vi "BMU参数读取-Auto.vi"(7 "Socket":dbl, 8 "CAN端口":u16(ring), 9 "设备索引号":u16(ring), 10 "CAN卡类型":u32(ring)=21, 11 "从板号":u8=1) -> (3 "成功?":bool)   [LabVIEW 2013] (continued)
                                n1192 = local write "均衡参数"(T18 {"充电结束电压(90%)"=0.0, "充电结束电压(91%)"=0.0, "充电结束电压(92%)"=0.0, "充电结束电压(93%)"=0.0, "充电结束电压(94%)"=0.0, "均衡计算-电压高阀值1级"=0.0, "均衡计算-电压高阀值2级"=0.0, "均衡计算-电压低阀值1级"=0.0, "均衡计算-电压低阀值2级"=0.0, "均衡计算-最低电压阀值"=0.0, "均衡停止-最低电压阀值"=0.0, "均衡计算-电压极差阀值"=0.0, "充电结束电压(95%)"=0.0, "充电结束电压(96%)"=0.0, "充电结束电压(97%)"=0.0, "充电结束电压(98%)"=0.0, "充电结束电压(99%)"=0.0, "充电结束电压(100%)"=0.0} ("均衡参数")) -> ()
                                }
                                frame "均衡阀值" {
                                w1936 = sgl 0.0 ("均衡计算-电压高阀值1级")
                                n1193 = local read "均衡参数"() -> (w1937:T18)
                                n1194 = Bundle By Name(cluster=w1937, "均衡计算-电压高阀值1级"=w1936, "均衡计算-电压高阀值2级"=w1936, "均衡计算-电压低阀值1级"=w1936, "均衡计算-电压低阀值2级"=w1936, "均衡计算-最低电压阀值"=w1936, "均衡停止-最低电压阀值"=w1936, "均衡计算-电压极差阀值"=w1936) -> (w1938:T18)
                                n1195 = local write "均衡参数"(w1938) -> ()
                                }
                                frame "充电结束电压" {
                                w1939 = sgl 0.0 ("均衡计算-电压高阀值1级")
                                n1196 = local read "均衡参数"() -> (w1940:T18)
                                n1197 = Bundle By Name(cluster=w1940, "充电结束电压(90%)"=w1939, "充电结束电压(91%)"=w1939, "充电结束电压(92%)"=w1939, "充电结束电压(93%)"=w1939, "充电结束电压(94%)"=w1939, "充电结束电压(95%)"=w1939, "充电结束电压(96%)"=w1939, "充电结束电压(97%)"=w1939, "充电结束电压(98%)"=w1939, "充电结束电压(99%)"=w1939, "充电结束电压(100%)"=w1939) -> (w1941:T18)
                                n1198 = local write "均衡参数"(w1941) -> ()
                                }
                                }
                              }
                            }
                          }
                          frame #1 {
                            w1942 = FALSE ("流控帧")
                            w1943 = TRUE ("流控帧 2")
                            n1199 = global write "EV05全局变量1.vi" "写入超时"(w1942) -> ()
                            n1200 = global write "EV05全局变量1.vi" "流控帧"(w1942) -> ()
                            n1201 = local write "写?"(w1942) -> ()
                            n1202 = local write "消除"(w1943) -> ()
                            n1203 = local write "控制1"(w1943) -> ()
                            n1204 = global write "EV05全局变量1.vi" "流控帧 2"(w1943) -> ()
                            n1205 = local write "写入超时"(w1942) -> ()
                            "流控帧" <- w1942
                            "流控帧 2" <- w1943
                          }
                          frame #2 {
                            n1206 = Wait Until Next ms Multiple(millisecond multiple=u32 300 ("毫秒倍数")) -> ()  [unwired: 1 out]
                          }
                          frame #3 {
                            n1207 = local read "设备索引号"() -> (w1946:u16)
                            n1208 = local read "CAN卡类型"() -> (w1947:u32)
                            n1209 = local read "CAN端口"() -> (w1945:u16)
                            n1210 = local write "命令序号"(w1950) -> ()
                            n1211 = stacked-sequence {
                              tunnel: w1951 -> [_ w1959]
                              tunnel: w1950 -> [_ w1958]
                              tunnel: w1949 -> [_ w1957]
                              tunnel: w1948 -> [_ w1956]
                              tunnel: w1947 -> [_ w1955]
                              tunnel: w1946 -> [_ w1954]
                              tunnel: w1945 -> [_ w1953]
                              frame #0 {
                              }
                              frame #1 {
                                n1212 = control-ref of="流控帧"() -> (w1952:refnum<vi>)
                                n1213 = call "多帧发送机制(EV05).vi"("can卡类型"=w1955, "设备索引号"=w1954, "CAN端口"=w1953, "命令"=w1959, "板号"=w1957, "命令序号"=w1958, "输入数据"=w1956, "流控帧"=w1952) -> ()  [unwired: 1 in, 11 out]
                              }
                            }
                          }
                          frame #4 {
                            n1214 = while {
                              tunnel: [w1964] -> w1961
                              tunnel: [w1962] -> w1960
                              i -> [w1967]
                              stop <- w1964 stop-if-true
                              n1215 = local read "强制终止读写标记"() -> (w1963:bool)
                              n1216 = local read "写入超时"() -> (w1962:bool)
                              n1217 = Greater Or Equal?(x=w1967, y=20) -> (x >= y?=w1965:bool)
                              n1218 = Compound Arithmetic op=OR(w1963, w1962, w1965) -> (w1964:bool)
                              n1219 = Wait Until Next ms Multiple(millisecond multiple=u32 100 ("毫秒倍数")) -> ()  [unwired: 1 out]
                            }
                          }
                          frame #5 {
                            n1220 = case shown="假" w1976 {
                              tunnel: w1975 -> [w1987 _]
                              tunnel: [w1982 w1999] -> w1974
                              tunnel: w1973 -> [w1981 _]
                              tunnel: w1972 -> [w1980 w1999]
                              tunnel: [w1979 w1998] -> w1969
                              tunnel: w1971 -> [w1978 _]
                              tunnel: w1970 -> [w1977 w1998]
                              frame False {
                                n1221 = local read "重试次数"() -> (w1986:u8)
                                n1222 = Increment(x=w1986) -> (x+1=w1985:u8)
                                n1223 = local write "重试次数"(w1985) -> ()
                                n1224 = Greater Or Equal?(x=w1985, y=u8 4) -> (x >= y?=w1984:bool)
                                n1225 = case shown="真" w1984 {
                                tunnel: w1987 -> [_ w1992]
                                tunnel: [w1989 w1991] -> w1982
                                tunnel: w1981 -> [w1989 _]
                                tunnel: w1980 -> [_ w1991]
                                tunnel: [w1988 w1990] -> w1979
                                tunnel: w1978 -> [w1988 _]
                                tunnel: w1977 -> [_ w1990]
                                frame False {
                                }
                                frame True {
                                n1226 = control-ref of="结果"() -> (w1994:refnum<vi>)
                                n1227 = Concatenate Strings(w1992, "     读取失败" ("字符串")) -> (w1996:string)
                                n1228 = Build Array(w1996) -> (w1993:string[])
                                n1229 = call "表格编辑.vi"("新元素/子数组"=w1993, "活动单元格:单元格背景色"=u32 16740749, "MCListbox引用句柄"=w1994) -> ()  [unwired: 9 out]
                                }
                                }
                              }
                              frame True {
                              }
                            }
                          }
                          frame #6 {
                            n1230 = And(x=w2001, y=w2003) -> (x .and. y?=w2002:bool)
                            n1231 = case shown="真" w2002 {
                              frame False {
                              }
                              frame True {
                                n1232 = local write "强制终止读写标记"(FALSE ("强制停止")) -> ()
                                n1233 = control-ref of="结果"() -> (w2006:refnum<vi>)
                                n1234 = Concatenate Strings("读取完成" ("字符串")) -> (w2008:string)
                                n1235 = Build Array(w2008) -> (w2005:string[])
                                n1236 = call "表格编辑.vi"("新元素/子数组"=w2005, "活动单元格:单元格背景色"=u32 21937, "MCListbox引用句柄"=w2006) -> ()  [unwired: 9 out]
                              }
                            }
                            n1237 = Wait (ms)(milliseconds to wait=u32 100 ("等待时间（毫秒）")) -> ()  [unwired: 1 out]
                          }
                        }
                      }
                    }
                  }
                  n1238 = local read "强制终止读写标记"() -> (w1773:bool)
                  n1239 = Or(x=w1773, y=w1772) -> (x .or. y?=w1770:bool)
                }
              }
            }
            frame #3 {
              n1240 = case shown="假" FALSE {
                tunnel: w2100 -> [w2101 _]
                frame False {
                  n1241 = case shown="\"从板\"" w2101 {
                    frame "主板", Default {
                      w2102 = "BCURESULT" ("section")
                      n1242 = global read "读配置文件全局.vi" "电池额定实际容量判定"() -> (w2124:bool)
                      n1243 = global read "读配置文件全局.vi" "电池充放电次数判定"() -> (w2113:bool)
                      n1244 = global read "读配置文件全局.vi" "加热控制参数判定"() -> (w2111:bool)
                      n1245 = global read "读配置文件全局.vi" "配置文件版本判定"() -> (w2123:bool)
                      n1246 = global read "读配置文件全局.vi" "充电控制参数判定"() -> (w2117:bool)
                      n1247 = global read "读配置文件全局.vi" "通道电压数判定"() -> (w2129:bool)
                      n1248 = global read "读配置文件全局.vi" "电压起始值判定"() -> (w2128:bool)
                      n1249 = global read "读配置文件全局.vi" "温度起始值判定"() -> (w2126:bool)
                      n1250 = global read "读配置文件全局.vi" "充放电安时判定"() -> (w2115:bool)
                      n1251 = global read "读配置文件全局.vi" "电池包组号判定"() -> (w2114:bool)
                      n1252 = global read "读配置文件全局.vi" "电池信息1判定"() -> (w2116:bool)
                      n1253 = global read "读配置文件全局.vi" "从板个数判定"() -> (w2132:bool)
                      n1254 = global read "读配置文件全局.vi" "产品编号判定"() -> (w2131:bool)
                      n1255 = global read "读配置文件全局.vi" "电压个数判定"() -> (w2130:bool)
                      n1256 = global read "读配置文件全局.vi" "温度个数判定"() -> (w2127:bool)
                      n1257 = global read "读配置文件全局.vi" "保险位置判定"() -> (w2125:bool)
                      n1258 = global read "读配置文件全局.vi" "一级故障判定"() -> (w2120:bool)
                      n1259 = global read "读配置文件全局.vi" "二级故障判定"() -> (w2119:bool)
                      n1260 = global read "读配置文件全局.vi" "三级故障判定"() -> (w2118:bool)
                      n1261 = global read "读配置文件全局.vi" "车牌号判定"() -> (w2122:bool)
                      n1262 = global read "读配置文件全局.vi" "SOH判定"() -> (w2121:bool)
                      n1263 = Build Array(w2132, w2131, w2130, w2129, w2128, w2127, w2126, w2125, w2124, w2123, w2122, w2121, w2120, w2119, w2118, w2117, w2116, w2115, w2114, w2113, w2111) -> (w2112:bool[])
                      n1264 = And Array Elements(Boolean array=w2112) -> (logical AND=w2133:bool)
                      n1265 = case shown="假" w2133 {
                        tunnel: w2112 -> [_ w2143]
                        tunnel: ["PASS" ("section") "FAIL" ("section")] -> w2103
                        frame True {
                          n1266 = control-ref of="结果"() -> (w2139:refnum<vi>)
                          n1267 = Build Array("全部判定成功!!!!!!!!") -> (w2140:string[])
                          n1268 = call "表格编辑.vi"("新元素/子数组"=w2140, "活动单元格:单元格背景色"=u32 6618880, "MCListbox引用句柄"=w2139) -> ()  [unwired: 9 out]
                          n1269 = local write "停止"(TRUE ("停止")) -> ()
                        }
                        frame False {
                          n1270 = stacked-sequence {
                            tunnel: w2143 -> [_ w2148]
                            frame #0 {
                              n1271 = control-ref of="结果"() -> (w2146:refnum<vi>)
                              n1272 = Build Array("全部判定失败!!!!!") -> (w2147:string[])
                              n1273 = call "表格编辑.vi"("新元素/子数组"=w2147, "活动单元格:单元格背景色"=u32 16711680, "MCListbox引用句柄"=w2146) -> ()  [unwired: 9 out]
                            }
                            frame #1 {
                              n1274 = for {
                                tunnel: w2148 -> [w2150] mode=indexing
                                i -> [w2149]
                                n1275 = case shown="17" w2149 {
                                tunnel: w2150 -> [w2151 w2156 w2161 w2166 w2171 w2176 w2181 w2186 w2191 w2196 w2201 w2206 w2211 w2216 w2221 w2226 w2231 w2236 w2241 w2246 w2251 _]
                                frame 0 {
                                n1276 = case shown="假" w2151 {
                                frame False {
                                n1277 = control-ref of="结果"() -> (w2154:refnum<vi>)
                                n1278 = Build Array("从板个数判定失败!") -> (w2155:string[])
                                n1279 = call "表格编辑.vi"("新元素/子数组"=w2155, "活动单元格:单元格背景色"=u32 16711680, "MCListbox引用句柄"=w2154) -> ()  [unwired: 9 out]
                                }
                                frame True {
                                }
                                }
                                }
                                frame 1 {
                                n1280 = case shown="假" w2156 {
                                frame False {
                                n1281 = control-ref of="结果"() -> (w2159:refnum<vi>)
                                n1282 = Build Array("产品编号判定失败!") -> (w2160:string[])
                                n1283 = call "表格编辑.vi"("新元素/子数组"=w2160, "活动单元格:单元格背景色"=u32 16711680, "MCListbox引用句柄"=w2159) -> ()  [unwired: 9 out]
                                }
                                frame True {
                                }
                                }
                                }
                                frame 2 {
                                n1284 = case shown="假" w2161 {
                                frame False {
                                n1285 = control-ref of="结果"() -> (w2164:refnum<vi>)
                                n1286 = Build Array("电压个数判定失败!") -> (w2165:string[])
                                n1287 = call "表格编辑.vi"("新元素/子数组"=w2165, "活动单元格:单元格背景色"=u32 16711680, "MCListbox引用句柄"=w2164) -> ()  [unwired: 9 out]
                                }
                                frame True {
                                }
                                }
                                }
                                frame 3 {
                                n1288 = case shown="假" w2166 {
                                frame False {
                                n1289 = control-ref of="结果"() -> (w2169:refnum<vi>)
                                n1290 = Build Array("通道电压数判定失败!") -> (w2170:string[])
                                n1291 = call "表格编辑.vi"("新元素/子数组"=w2170, "活动单元格:单元格背景色"=u32 16711680, "MCListbox引用句柄"=w2169) -> ()  [unwired: 9 out]
                                }
                                frame True {
                                }
                                }
                                }
                                frame 4 {
                                n1292 = case shown="假" w2171 {
                                frame False {
                                n1293 = control-ref of="结果"() -> (w2174:refnum<vi>)
                                n1294 = Build Array("电压起始值判定失败!") -> (w2175:string[])
                                n1295 = call "表格编辑.vi"("新元素/子数组"=w2175, "活动单元格:单元格背景色"=u32 16711680, "MCListbox引用句柄"=w2174) -> ()  [unwired: 9 out]
                                }
                                frame True {
                                }
                                }
                                }
                                frame 5 {
                                n1296 = case shown="假" w2176 {
                                frame False {
                                n1297 = control-ref of="结果"() -> (w2179:refnum<vi>)
                                n1298 = Build Array("温度个数判定失败!") -> (w2180:string[])
                                n1299 = call "表格编辑.vi"("新元素/子数组"=w2180, "活动单元格:单元格背景色"=u32 16711680, "MCListbox引用句柄"=w2179) -> ()  [unwired: 9 out]
                                }
                                frame True {
                                }
                                }
                                }
                                frame 6 {
                                n1300 = case shown="假" w2181 {
                                frame False {
                                n1301 = control-ref of="结果"() -> (w2184:refnum<vi>)
                                n1302 = Build Array("温度起始值判定失败!") -> (w2185:string[])
                                n1303 = call "表格编辑.vi"("新元素/子数组"=w2185, "活动单元格:单元格背景色"=u32 16711680, "MCListbox引用句柄"=w2184) -> ()  [unwired: 9 out]
                                }
                                frame True {
                                }
                                }
                                }
                                frame 7 {
                                n1304 = case shown="假" w2186 {
                                frame False {
                                n1305 = control-ref of="结果"() -> (w2189:refnum<vi>)
                                n1306 = Build Array("保险位置判定失败!") -> (w2190:string[])
                                n1307 = call "表格编辑.vi"("新元素/子数组"=w2190, "活动单元格:单元格背景色"=u32 16711680, "MCListbox引用句柄"=w2189) -> ()  [unwired: 9 out]
                                }
                                frame True {
                                }
                                }
                                }
                                frame 8 {
                                n1308 = case shown="假" w2191 {
                                frame False {
                                n1309 = control-ref of="结果"() -> (w2194:refnum<vi>)
                                n1310 = Build Array("电池额定实际容量判定失败!") -> (w2195:string[])
                                n1311 = call "表格编辑.vi"("新元素/子数组"=w2195, "活动单元格:单元格背景色"=u32 16711680, "MCListbox引用句柄"=w2194) -> ()  [unwired: 9 out]
                                }
                                frame True {
                                }
                                }
                                }
                                frame 9 {
                                n1312 = case shown="假" w2196 {
                                frame False {
                                n1313 = control-ref of="结果"() -> (w2199:refnum<vi>)
                                n1314 = Build Array("配置文件版本判定失败!") -> (w2200:string[])
                                n1315 = call "表格编辑.vi"("新元素/子数组"=w2200, "活动单元格:单元格背景色"=u32 16711680, "MCListbox引用句柄"=w2199) -> ()  [unwired: 9 out]
                                }
                                frame True {
                                }
                                }
                                }
                                frame 10 {
                                n1316 = case shown="假" w2201 {
                                frame False {
                                n1317 = control-ref of="结果"() -> (w2204:refnum<vi>)
                                n1318 = Build Array("车牌号判定失败!") -> (w2205:string[])
                                n1319 = call "表格编辑.vi"("新元素/子数组"=w2205, "活动单元格:单元格背景色"=u32 16711680, "MCListbox引用句柄"=w2204) -> ()  [unwired: 9 out]
                                }
                                frame True {
                                }
                                }
                                }
                                frame 11 {
                                n1320 = case shown="假" w2206 {
                                frame False {
                                n1321 = control-ref of="结果"() -> (w2209:refnum<vi>)
                                n1322 = Build Array("SOH判定失败!") -> (w2210:string[])
                                n1323 = call "表格编辑.vi"("新元素/子数组"=w2210, "活动单元格:单元格背景色"=u32 16711680, "MCListbox引用句柄"=w2209) -> ()  [unwired: 9 out]
                                }
                                frame True {
                                }
                                }
                                }
                                frame 12 {
                                n1324 = case shown="假" w2211 {
                                frame False {
                                n1325 = control-ref of="结果"() -> (w2214:refnum<vi>)
                                n1326 = Build Array("一级故障阀值判定失败!") -> (w2215:string[])
                                n1327 = call "表格编辑.vi"("新元素/子数组"=w2215, "活动单元格:单元格背景色"=u32 16711680, "MCListbox引用句柄"=w2214) -> ()  [unwired: 9 out]
                                }
                                frame True {
                                }
                                }
                                }
                                frame 13 {
                                n1328 = case shown="假" w2216 {
                                frame False {
                                n1329 = control-ref of="结果"() -> (w2219:refnum<vi>)
                                n1330 = Build Array("二级故障阀值判定失败!") -> (w2220:string[])
                                n1331 = call "表格编辑.vi"("新元素/子数组"=w2220, "活动单元格:单元格背景色"=u32 16711680, "MCListbox引用句柄"=w2219) -> ()  [unwired: 9 out]
                                }
                                frame True {
                                }
                                }
                                }
                                frame 14 {
                                n1332 = case shown="假" w2221 {
                                frame False {
                                n1333 = control-ref of="结果"() -> (w2224:refnum<vi>)
                                n1334 = Build Array("三级故障阀值判定失败!") -> (w2225:string[])
                                n1335 = call "表格编辑.vi"("新元素/子数组"=w2225, "活动单元格:单元格背景色"=u32 16711680, "MCListbox引用句柄"=w2224) -> ()  [unwired: 9 out]
                                }
                                frame True {
                                }
                                }
                                }
                                frame 15 {
                                n1336 = case shown="假" w2226 {
                                frame False {
                                n1337 = control-ref of="结果"() -> (w2229:refnum<vi>)
                                n1338 = Build Array("充电控制参数判定失败!") -> (w2230:string[])
                                n1339 = call "表格编辑.vi"("新元素/子数组"=w2230, "活动单元格:单元格背景色"=u32 16711680, "MCListbox引用句柄"=w2229) -> ()  [unwired: 9 out]
                                }
                                frame True {
                                }
                                }
                                }
                                frame 16 {
                                n1340 = case shown="假" w2231 {
                                frame False {
                                n1341 = control-ref of="结果"() -> (w2234:refnum<vi>)
                                n1342 = Build Array("电池信息1判定失败!") -> (w2235:string[])
                                n1343 = call "表格编辑.vi"("新元素/子数组"=w2235, "活动单元格:单元格背景色"=u32 16711680, "MCListbox引用句柄"=w2234) -> ()  [unwired: 9 out]
                                }
                                frame True {
                                }
                                }
                                }
                                frame 17 {
                                n1344 = case shown="假" w2236 {
                                frame False {
                                n1345 = control-ref of="结果"() -> (w2239:refnum<vi>)
                                n1346 = Build Array("充放电安时判定失败!") -> (w2240:string[])
                                n1347 = call "表格编辑.vi"("新元素/子数组"=w2240, "活动单元格:单元格背景色"=u32 16711680, "MCListbox引用句柄"=w2239) -> ()  [unwired: 9 out]
                                }
                                frame True {
                                }
                                }
                                }
                                frame 18 {
                                n1348 = case shown="假" w2241 {
                                frame False {
                                n1349 = control-ref of="结果"() -> (w2244:refnum<vi>)
                                n1350 = Build Array("电池包组号判定失败!") -> (w2245:string[])
                                n1351 = call "表格编辑.vi"("新元素/子数组"=w2245, "活动单元格:单元格背景色"=u32 16711680, "MCListbox引用句柄"=w2244) -> ()  [unwired: 9 out]
                                }
                                frame True {
                                }
                                }
                                }
                                frame 19 {
                                n1352 = case shown="假" w2246 {
                                frame False {
                                n1353 = control-ref of="结果"() -> (w2249:refnum<vi>)
                                n1354 = Build Array("电池充放电次数判定失败!") -> (w2250:string[])
                                n1355 = call "表格编辑.vi"("新元素/子数组"=w2250, "活动单元格:单元格背景色"=u32 16711680, "MCListbox引用句柄"=w2249) -> ()  [unwired: 9 out]
                                }
                                frame True {
                                }
                                }
                                }
                                frame 20 {
                                n1356 = case shown="假" w2251 {
                                frame False {
                                n1357 = control-ref of="结果"() -> (w2254:refnum<vi>)
                                n1358 = Build Array("加热控制参数判定失败!") -> (w2255:string[])
                                n1359 = call "表格编辑.vi"("新元素/子数组"=w2255, "活动单元格:单元格背景色"=u32 16711680, "MCListbox引用句柄"=w2254) -> ()  [unwired: 9 out]
                                }
                                frame True {
                                }
                                }
                                }
                                frame 99, Default {
                                }
                                }
                              }
                            }
                          }
                          n1360 = local write "停止"(TRUE ("停止")) -> ()
                        }
                      }
                      n1361 = call <vilib>:"Open Config Data.vi"("create file if necessary (T)"=FALSE, "configuration file path"=path "D:/BlueWay/configresult.ini") -> ("error out"=w2107:errorcluster, "refnum"=w2108:T26)  [unwired: 7 in, 1 out]
                      n1362 = call-poly <vilib>:"Write Key.vi"("section"=w2102, "error in (no error)"=w2107, "value"=w2103, "key"=w2102, "refnum"=w2108) -> ("error out"=w2105:errorcluster, "refnum out"=w2106:T26)  [unwired: 4 in, 1 out]
                      n1363 = call <vilib>:"Close Config Data.vi"("error in (no error)"=w2105, "refnum"=w2106) -> ("error out"=w2104:errorcluster)  [unwired: 8 in, 1 out]
                      n1364 = flat-sequence {
                        tunnel: w2104 -> [_]
                        frame #0 {
                          n1365 = disable-structure shown="启用" {
                            frame Enabled {
                              n1366 = Quit LabVIEW(quit? (T)=TRUE ("退出？(T)")) -> ()
                            }
                            frame Disabled {
                            }
                          }
                        }
                      }
                    }
                    frame "从板" {
                      w2261 = "BMURESULT" ("section")
                      n1367 = global read "读配置文件全局2.vi" "三级故障判定"() -> (w2269:bool)
                      n1368 = global read "读配置文件全局2.vi" "电压起始值判定"() -> (w2275:bool)
                      n1369 = global read "读配置文件全局2.vi" "通道电压判定"() -> (w2274:bool)
                      n1370 = global read "读配置文件全局2.vi" "保险位置判定"() -> (w2273:bool)
                      n1371 = global read "读配置文件全局2.vi" "温度起始值判定"() -> (w2272:bool)
                      n1372 = global read "读配置文件全局2.vi" "一级故障判定"() -> (w2271:bool)
                      n1373 = global read "读配置文件全局2.vi" "二级故障判定"() -> (w2270:bool)
                      n1374 = global read "读配置文件全局2.vi" "从板号判定"() -> (w2276:bool)
                      n1375 = control-ref of="BMU读取结果"() -> (w2258:refnum<vi>)
                      n1376 = Build Array(w2276, w2275, w2274, w2273, w2272, w2271, w2270, w2269) -> ()  [unwired: 1 out]
                      n1377 = property class="Clust (严格)"(reference=w2258) -> ("Value"=w2257:T8)  [unwired: 1 in, 2 out]
                      n1378 = Cluster To Array(cluster=w2257) -> (array=w2256:bool[])
                      n1379 = And Array Elements(Boolean array=w2256) -> (logical AND=w2277:bool)
                      n1380 = case shown="假" w2277 {
                        tunnel: w2256 -> [_ w2287]
                        tunnel: ["PASS" ("section") "FAIL" ("section")] -> w2260
                        tunnel: [TRUE ("成功?") FALSE ("成功?")] -> w2259
                        frame True {
                          n1381 = control-ref of="结果"() -> (w2283:refnum<vi>)
                          n1382 = Build Array("读取判定成功!!!!!!!!") -> (w2284:string[])
                          n1383 = call "表格编辑.vi"("新元素/子数组"=w2284, "活动单元格:单元格背景色"=u32 6618880, "MCListbox引用句柄"=w2283) -> ()  [unwired: 9 out]
                        }
                        frame False {
                          n1384 = stacked-sequence {
                            tunnel: w2287 -> [_ w2292]
                            frame #0 {
                              n1385 = control-ref of="结果"() -> (w2290:refnum<vi>)
                              n1386 = Build Array("读取判定失败!!!!!") -> (w2291:string[])
                              n1387 = call "表格编辑.vi"("新元素/子数组"=w2291, "活动单元格:单元格背景色"=u32 16711680, "MCListbox引用句柄"=w2290) -> ()  [unwired: 9 out]
                            }
                            frame #1 {
                              n1388 = for {
                                tunnel: w2292 -> [w2293] mode=indexing
                                i -> [w2294]
                                n1389 = case shown="3" w2294 {
                                tunnel: w2293 -> [w2295 w2300 w2305 w2310 w2315 w2320 w2325 w2330 w2335 _]
                                frame 0 {
                                n1390 = case shown="假" w2295 {
                                frame False {
                                n1391 = control-ref of="结果"() -> (w2298:refnum<vi>)
                                n1392 = Build Array("从板号判定失败!") -> (w2299:string[])
                                n1393 = call "表格编辑.vi"("新元素/子数组"=w2299, "活动单元格:单元格背景色"=u32 16711680, "MCListbox引用句柄"=w2298) -> ()  [unwired: 9 out]
                                }
                                frame True {
                                }
                                }
                                }
                                frame 1 {
                                n1394 = case shown="假" w2300 {
                                frame False {
                                n1395 = control-ref of="结果"() -> (w2303:refnum<vi>)
                                n1396 = Build Array("电压起始值判定失败!") -> (w2304:string[])
                                n1397 = call "表格编辑.vi"("新元素/子数组"=w2304, "活动单元格:单元格背景色"=u32 16711680, "MCListbox引用句柄"=w2303) -> ()  [unwired: 9 out]
                                }
                                frame True {
                                }
                                }
                                }
                                frame 2 {
                                n1398 = case shown="假" w2305 {
                                frame False {
                                n1399 = control-ref of="结果"() -> (w2308:refnum<vi>)
                                n1400 = Build Array("通道电压节数判定失败!") -> (w2309:string[])
                                n1401 = call "表格编辑.vi"("新元素/子数组"=w2309, "活动单元格:单元格背景色"=u32 16711680, "MCListbox引用句柄"=w2308) -> ()  [unwired: 9 out]
                                }
                                frame True {
                                }
                                }
                                }
                                frame 3 {
                                n1402 = case shown="假" w2310 {
                                frame False {
                                n1403 = control-ref of="结果"() -> (w2313:refnum<vi>)
                                n1404 = Build Array("保险位置判定失败!") -> (w2314:string[])
                                n1405 = call "表格编辑.vi"("新元素/子数组"=w2314, "活动单元格:单元格背景色"=u32 16711680, "MCListbox引用句柄"=w2313) -> ()  [unwired: 9 out]
                                }
                                frame True {
                                }
                                }
                                }
                                frame 4 {
                                n1406 = case shown="假" w2315 {
                                frame False {
                                n1407 = control-ref of="结果"() -> (w2318:refnum<vi>)
                                n1408 = Build Array("温度起始值判定失败!") -> (w2319:string[])
                                n1409 = call "表格编辑.vi"("新元素/子数组"=w2319, "活动单元格:单元格背景色"=u32 16711680, "MCListbox引用句柄"=w2318) -> ()  [unwired: 9 out]
                                }
                                frame True {
                                }
                                }
                                }
                                frame 5 {
                                n1410 = case shown="假" w2320 {
                                frame False {
                                n1411 = control-ref of="结果"() -> (w2323:refnum<vi>)
                                n1412 = Build Array("一级故障判定失败!") -> (w2324:string[])
                                n1413 = call "表格编辑.vi"("新元素/子数组"=w2324, "活动单元格:单元格背景色"=u32 16711680, "MCListbox引用句柄"=w2323) -> ()  [unwired: 9 out]
                                }
                                frame True {
                                }
                                }
                                }
                                frame 6 {
                                n1414 = case shown="假" w2325 {
                                frame False {
                                n1415 = control-ref of="结果"() -> (w2328:refnum<vi>)
                                n1416 = Build Array("二级故障判定失败!") -> (w2329:string[])
                                n1417 = call "表格编辑.vi"("新元素/子数组"=w2329, "活动单元格:单元格背景色"=u32 16711680, "MCListbox引用句柄"=w2328) -> ()  [unwired: 9 out]
                                }
                                frame True {
                                }
                                }
                                }
                                frame 7 {
                                n1418 = case shown="假" w2330 {
                                frame False {
                                n1419 = control-ref of="结果"() -> (w2333:refnum<vi>)
                                n1420 = Build Array("三级故障判定失败!") -> (w2334:string[])
                                n1421 = call "表格编辑.vi"("新元素/子数组"=w2334, "活动单元格:单元格背景色"=u32 16711680, "MCListbox引用句柄"=w2333) -> ()  [unwired: 9 out]
                                }
                                frame True {
                                }
                                }
                                }
                                frame 8 {
                                n1422 = case shown="假" w2335 {
                                frame False {
                                n1423 = control-ref of="结果"() -> (w2338:refnum<vi>)
                                n1424 = Build Array("加热控制参数判定失败!") -> (w2339:string[])
                                n1425 = call "表格编辑.vi"("新元素/子数组"=w2339, "活动单元格:单元格背景色"=u32 16711680, "MCListbox引用句柄"=w2338) -> ()  [unwired: 9 out]
                                }
                                frame True {
                                }
                                }
                                }
                                frame 99, Default {
                                }
                                }
                              }
                            }
                          }
                        }
                      }
                      "成功?" <- w2259
                      n1426 = call <vilib>:"Open Config Data.vi"("create file if necessary (T)"=FALSE, "configuration file path"=path "D:/BlueWay/configresult.ini") -> ("error out"=w2265:errorcluster, "refnum"=w2266:T26)  [unwired: 7 in, 1 out]
                      n1427 = call-poly <vilib>:"Write Key.vi"("section"=w2261, "error in (no error)"=w2265, "value"=w2260, "key"=w2261, "refnum"=w2266) -> ("error out"=w2263:errorcluster, "refnum out"=w2264:T26)  [unwired: 4 in, 1 out]
                      n1428 = call <vilib>:"Close Config Data.vi"("error in (no error)"=w2263, "refnum"=w2264) -> ("error out"=w2262:errorcluster)  [unwired: 8 in, 1 out]
                      n1429 = stacked-sequence {
                        tunnel: w2262 -> [_]
                        frame #0 {
                          n1430 = local write "停止"(TRUE ("退出？(T)")) -> ()
                        }
                      }
                    }
                  }
                }
                frame True {
                }
              }
            }
          }
          n1431 = stacked-sequence {
            tunnel: w1101 -> [_]
            frame #0 {
              n1432 = local write "强制终止读写标记"(FALSE ("强制停止")) -> ()
            }
          }
          "重试次数" <- u8 0 ("重试次数")
        }
        frame "开启均衡" {
          n1433 = local read "从板板号"() -> (w2340:u8)
          n1434 = stacked-sequence {
            tunnel: 133 -> [_ w2366 _ _]
            tunnel: w2340 -> [_ _ _ _]
            frame #0 {
              w2350 = u8 0 items=["Normal", "Listen Only"] ("工作方式")
              w2349 = u8 1 items=["Dual Filter", "Single Filter"] ("滤波方式")
              n1435 = global write "EV05全局变量1.vi" "读取超时"(FALSE ("读取超时")) -> ()
              n1436 = global write "EV05全局变量1.vi" "流控帧 2"(TRUE ("流控帧 2")) -> ()
              n1437 = local write "写?"(TRUE ("写?")) -> ()
              n1438 = local read "设备索引号"() -> (w2345:u16)
              n1439 = local read "CAN卡类型"() -> (w2344:u32)
              n1440 = local read "CAN端口"() -> (w2346:u16)
              n1441 = local write "控制1"(TRUE ("控制1")) -> ()
              n1442 = local write "消除"(TRUE ("消除")) -> ()
              n1443 = global write "EV05全局变量1.vi" "流控帧"(FALSE ("流控帧")) -> ()
              n1444 = call "CAN_Init-8.6.vi"("CAN卡类型"=w2344, "设备索引号"=w2345, "CAN端口"=w2346, "操作类型"=enum16{"初始化CAN", "关闭CAN"}."初始化CAN", "滤波方式"=w2349, "Accept Code"=u32 606601216, "簇"=T22 {"打开CAN"=FALSE, "初始化CAN"=TRUE, "开始CAN"=TRUE, "重启"=FALSE, "关闭CAN"=FALSE}, "Mask Code"=u32 524287 ("Accept Code"), "工作方式"=w2350, "是否滤波"=TRUE, "滤波选择"=T21 {"fiter_mode"=1, "fiter_endid"=75825152, "fiter_startid"=75890687}) -> ()  [unwired: 3 in, 6 out]
              n1445 = Wait Until Next ms Multiple(millisecond multiple=u32 20 ("毫秒倍数")) -> ()  [unwired: 1 out]
            }
            frame #1 {
              n1446 = local write "命令"(w2366) -> ()
              n1447 = call "ID组合.vi"("SA(4)"=0 ("PDU(1)"), "PS(3)"=63 ("PDU(1)"), "PF(2)"=w2366, "PDU(1)"=4) -> ("ID"=w2365:i32)  [unwired: 7 out]
              n1448 = local read "均衡类型选择"() -> (w2362:enum16{"放电均衡", "充电均衡", "充放电均衡"})
              n1449 = local read "设备索引号"() -> (w2371:u16)
              n1450 = local read "CAN卡类型"() -> (w2372:u32)
              n1451 = local read "CAN端口"() -> (w2370:u16)
              n1452 = local write "命令序号"(2) -> ()
              n1453 = Add(x=w2362, y=1) -> (x+y=w2360:i32)
              n1454 = Build Array(2, 2, w2360) -> (w2373:i32[])
              n1455 = call "transmit-8.6.vi"("can卡类型"=w2372, "设备索引号"=w2371, "CAN端口"=w2370, "ID"=w2365, "SendType"=u8 0, "Data"=w2373) -> ()  [unwired: 3 in, 11 out]
            }
            frame #2 {
              n1456 = Wait Until Next ms Multiple(millisecond multiple=u32 1000 ("毫秒倍数")) -> ()  [unwired: 1 out]
            }
            frame #3 {
              w2381 = u8 0 items=["Normal", "Listen Only"] ("工作方式")
              w2382 = u8 1 items=["Dual Filter", "Single Filter"] ("滤波方式")
              n1457 = global write "EV05全局变量1.vi" "流控帧 2"(FALSE ("流控帧 2")) -> ()
              n1458 = local read "CAN卡类型"() -> (w2387:u32)
              n1459 = local read "设备索引号"() -> (w2386:u16)
              n1460 = local read "CAN端口"() -> (w2385:u16)
              n1461 = local write "控制1"(FALSE ("控制1")) -> ()
              n1462 = local write "消除"(FALSE ("消除")) -> ()
              n1463 = call <vilib>:"Unset Busy.vi"() -> ()  [unwired: 2 in, 10 out]
              n1464 = call "CAN_Init-8.6.vi"("CAN卡类型"=w2387, "设备索引号"=w2386, "CAN端口"=w2385, "操作类型"=enum16{"初始化CAN", "关闭CAN"}."初始化CAN", "滤波方式"=w2382, "Accept Code"=u32 3221225472, "簇"=T22 {"打开CAN"=FALSE, "初始化CAN"=TRUE, "开始CAN"=TRUE, "重启"=FALSE, "关闭CAN"=FALSE}, "Mask Code"=u32 1073741823 ("Accept Code"), "工作方式"=w2381, "是否滤波"=TRUE, "滤波选择"=T21 {"fiter_mode"=1, "fiter_endid"=402653184, "fiter_startid"=419430399}) -> ()  [unwired: 3 in, 6 out]
            }
          }
        }
        frame "关闭均衡" {
          n1465 = local read "从板板号"() -> (w2391:u8)
          n1466 = stacked-sequence {
            tunnel: 133 -> [_ w2415 _ _]
            tunnel: w2391 -> [_ _ _ _]
            frame #0 {
              w2401 = u8 0 items=["Normal", "Listen Only"] ("工作方式")
              w2400 = u8 1 items=["Dual Filter", "Single Filter"] ("滤波方式")
              n1467 = global write "EV05全局变量1.vi" "读取超时"(FALSE ("读取超时")) -> ()
              n1468 = global write "EV05全局变量1.vi" "流控帧 2"(TRUE ("流控帧 2")) -> ()
              n1469 = local write "写?"(TRUE ("写?")) -> ()
              n1470 = local read "设备索引号"() -> (w2396:u16)
              n1471 = local read "CAN卡类型"() -> (w2395:u32)
              n1472 = local read "CAN端口"() -> (w2397:u16)
              n1473 = local write "控制1"(TRUE ("控制1")) -> ()
              n1474 = global write "EV05全局变量1.vi" "流控帧"(FALSE ("流控帧")) -> ()
              n1475 = local write "消除"(TRUE ("消除")) -> ()
              n1476 = call "CAN_Init-8.6.vi"("CAN卡类型"=w2395, "设备索引号"=w2396, "CAN端口"=w2397, "操作类型"=enum16{"初始化CAN", "关闭CAN"}."初始化CAN", "滤波方式"=w2400, "Accept Code"=u32 606601216, "簇"=T22 {"打开CAN"=FALSE, "初始化CAN"=TRUE, "开始CAN"=TRUE, "重启"=FALSE, "关闭CAN"=FALSE}, "Mask Code"=u32 524287 ("Accept Code"), "工作方式"=w2401, "是否滤波"=TRUE, "滤波选择"=T21 {"fiter_mode"=1, "fiter_endid"=75825152, "fiter_startid"=75890687}) -> ()  [unwired: 3 in, 6 out]
              n1477 = Wait Until Next ms Multiple(millisecond multiple=u32 20 ("毫秒倍数")) -> ()  [unwired: 1 out]
            }
            frame #1 {
              n1478 = local write "命令"(w2415) -> ()
              n1479 = call "ID组合.vi"("SA(4)"=0 ("PDU(1)"), "PS(3)"=63 ("PDU(1)"), "PF(2)"=w2415, "PDU(1)"=4) -> ("ID"=w2414:i32)  [unwired: 7 out]
              n1480 = local read "均衡类型选择"() -> (w2425:enum16{"放电均衡", "充电均衡", "充放电均衡"})
              n1481 = local write "命令序号"(3) -> ()
              n1482 = local read "设备索引号"() -> (w2420:u16)
              n1483 = local read "CAN卡类型"() -> (w2421:u32)
              n1484 = local read "CAN端口"() -> (w2419:u16)
              n1485 = Add(x=w2425, y=1) -> (x+y=w2423:i32)
              n1486 = Build Array(2, 3, w2423) -> (w2422:i32[])
              n1487 = call "transmit-8.6.vi"("can卡类型"=w2421, "设备索引号"=w2420, "CAN端口"=w2419, "ID"=w2414, "SendType"=u8 0, "Data"=w2422) -> ()  [unwired: 3 in, 11 out]
            }
            frame #2 {
              n1488 = Wait Until Next ms Multiple(millisecond multiple=u32 1000 ("毫秒倍数")) -> ()  [unwired: 1 out]
            }
            frame #3 {
              w2432 = u8 0 items=["Normal", "Listen Only"] ("工作方式")
              w2433 = u8 1 items=["Dual Filter", "Single Filter"] ("滤波方式")
              n1489 = local read "设备索引号"() -> (w2437:u16)
              n1490 = local read "CAN卡类型"() -> (w2438:u32)
              n1491 = global write "EV05全局变量1.vi" "流控帧 2"(FALSE ("流控帧 2")) -> ()
              n1492 = local read "CAN端口"() -> (w2436:u16)
              n1493 = local write "控制1"(FALSE ("控制1")) -> ()
              n1494 = local write "消除"(FALSE ("消除")) -> ()
              n1495 = call "CAN_Init-8.6.vi"("CAN卡类型"=w2438, "设备索引号"=w2437, "CAN端口"=w2436, "操作类型"=enum16{"初始化CAN", "关闭CAN"}."初始化CAN", "滤波方式"=w2433, "Accept Code"=u32 3221225472, "簇"=T22 {"打开CAN"=FALSE, "初始化CAN"=TRUE, "开始CAN"=TRUE, "重启"=FALSE, "关闭CAN"=FALSE}, "Mask Code"=u32 1073741823 ("Accept Code"), "工作方式"=w2432, "是否滤波"=TRUE, "滤波选择"=T21 {"fiter_mode"=1, "fiter_endid"=402653184, "fiter_startid"=419430399}) -> ()  [unwired: 3 in, 6 out]
              n1496 = call <vilib>:"Unset Busy.vi"() -> ()  [unwired: 2 in, 10 out]
            }
          }
        }
        frame "强制均衡" {
          n1497 = local read "从板板号"() -> (w2442:u8)
          n1498 = stacked-sequence {
            tunnel: 133 -> [_ w2473 _ _]
            tunnel: w2442 -> [_ _ _ _]
            frame #0 {
              w2452 = u8 0 items=["Normal", "Listen Only"] ("工作方式")
              w2451 = u8 1 items=["Dual Filter", "Single Filter"] ("滤波方式")
              n1499 = global write "EV05全局变量1.vi" "读取超时"(FALSE ("读取超时")) -> ()
              n1500 = global write "EV05全局变量1.vi" "流控帧 2"(TRUE ("流控帧 2")) -> ()
              n1501 = local write "写?"(TRUE ("写?")) -> ()
              n1502 = local read "设备索引号"() -> (w2447:u16)
              n1503 = local read "CAN卡类型"() -> (w2446:u32)
              n1504 = local write "控制1"(TRUE ("控制1")) -> ()
              n1505 = local read "CAN端口"() -> (w2448:u16)
              n1506 = local write "消除"(TRUE ("消除")) -> ()
              n1507 = global write "EV05全局变量1.vi" "流控帧"(FALSE ("流控帧")) -> ()
              n1508 = call "CAN_Init-8.6.vi"("CAN卡类型"=w2446, "设备索引号"=w2447, "CAN端口"=w2448, "操作类型"=enum16{"初始化CAN", "关闭CAN"}."初始化CAN", "滤波方式"=w2451, "Accept Code"=u32 606601216, "簇"=T22 {"打开CAN"=FALSE, "初始化CAN"=TRUE, "开始CAN"=TRUE, "重启"=FALSE, "关闭CAN"=FALSE}, "Mask Code"=u32 524287 ("Accept Code"), "工作方式"=w2452, "是否滤波"=TRUE, "滤波选择"=T21 {"fiter_mode"=1, "fiter_endid"=75825152, "fiter_startid"=75890687}) -> ()  [unwired: 3 in, 6 out]
              n1509 = Wait Until Next ms Multiple(millisecond multiple=u32 20 ("毫秒倍数")) -> ()  [unwired: 1 out]
            }
            frame #1 {
              n1510 = local read "强制类型"() -> (w2479:enum16{"全通道开启", "单通道开启", "清待均衡时间"})
              n1511 = case shown="\"清待均衡时间\"" w2479 {
                tunnel: [250 252 254] -> w2469
                tunnel: [_ w2498 _] -> w2468
                tunnel: [_ w2497 _] -> w2467
                tunnel: [_ w2488 _] -> w2466
                tunnel: [_ w2481 _] -> w2465
                frame "全通道开启", Default {
                }
                frame "单通道开启" {
                  n1512 = local read "均衡类型选择"() -> (w2496:enum16{"放电均衡", "充电均衡", "充放电均衡"})
                  n1513 = local read "均衡位置"() -> (w2491:u16)
                  n1514 = case shown="\"放电均衡\", 默认" w2496 {
                    tunnel: [0 1] -> w2495
                    frame "放电均衡", Default {
                    }
                    frame "充电均衡" {
                    }
                  }
                  n1515 = Multiply(x="均衡时间", y=6.0) -> (x*y=w2483:dbl)
                  n1516 = Quotient & Remainder(x=w2483, y=256.0) -> (x-y*floor(x/y)=w2481:dbl, floor(x/y)=w2482:dbl)
                  n1517 = call "二进制解析-8.6.vi"("索引"=1, "数值"=w2495) -> ("低位子数组"=w2486:i32[])  [unwired: 1 in, 2 out]
                  n1518 = Quotient & Remainder(x=w2491, y=256.0) -> (x-y*floor(x/y)=w2497:dbl, floor(x/y)=w2498:dbl)
                  n1519 = call "二进制解析-8.6.vi"("索引"=8, "数值"=w2482) -> ("低位子数组"=w2487:i32[])  [unwired: 1 in, 2 out]
                  n1520 = Replace Array Subset(array=w2487, new element=w2486, index=0 ("索引")) -> (w2484:i32[])
                  n1521 = call "数值二进制转十进制-8.6.vi"("子数组"=w2484) -> ("十进制数值"=w2488:i32)  [unwired: 4 in]
                }
                frame "清待均衡时间" {
                }
              }
              n1522 = local write "命令"(w2473) -> ()
              n1523 = call "ID组合.vi"("SA(4)"=0 ("PDU(1)"), "PS(3)"=63 ("PDU(1)"), "PF(2)"=w2473, "PDU(1)"=4) -> ("ID"=w2472:i32)  [unwired: 7 out]
              n1524 = local read "设备索引号"() -> (w2476:u16)
              n1525 = local read "CAN卡类型"() -> (w2477:u32)
              n1526 = local read "CAN端口"() -> (w2475:u16)
              n1527 = local write "命令序号"(w2469) -> ()
              n1528 = Build Array(6, 4, w2469, w2468, w2467, w2466, w2465) -> (w2478:dbl[])
              n1529 = call "transmit-8.6.vi"("can卡类型"=w2477, "设备索引号"=w2476, "CAN端口"=w2475, "ID"=w2472, "SendType"=u8 0, "Data"=w2478) -> ()  [unwired: 3 in, 11 out]
            }
            frame #2 {
              n1530 = Wait Until Next ms Multiple(millisecond multiple=u32 1000 ("毫秒倍数")) -> ()  [unwired: 1 out]
            }
            frame #3 {
              w2512 = u8 0 items=["Normal", "Listen Only"] ("工作方式")
              w2511 = u8 1 items=["Dual Filter", "Single Filter"] ("滤波方式")
              n1531 = global write "EV05全局变量1.vi" "流控帧 2"(FALSE ("流控帧 2")) -> ()
              n1532 = local write "控制1"(FALSE ("控制1")) -> ()
              n1533 = local read "设备索引号"() -> (w2507:u16)
              n1534 = local read "CAN卡类型"() -> (w2506:u32)
              n1535 = local write "消除"(FALSE ("消除")) -> ()
              n1536 = local read "CAN端口"() -> (w2508:u16)
              n1537 = call <vilib>:"Unset Busy.vi"() -> ()  [unwired: 2 in, 10 out]
              n1538 = call "CAN_Init-8.6.vi"("CAN卡类型"=w2506, "设备索引号"=w2507, "CAN端口"=w2508, "操作类型"=enum16{"初始化CAN", "关闭CAN"}."初始化CAN", "滤波方式"=w2511, "Accept Code"=u32 3221225472, "簇"=T22 {"打开CAN"=FALSE, "初始化CAN"=TRUE, "开始CAN"=TRUE, "重启"=FALSE, "关闭CAN"=FALSE}, "Mask Code"=u32 1073741823 ("Accept Code"), "工作方式"=w2512, "是否滤波"=TRUE, "滤波选择"=T21 {"fiter_mode"=1, "fiter_endid"=402653184, "fiter_startid"=419430399}) -> ()  [unwired: 3 in, 6 out]
            }
          }
        }
        frame "项目软件版本读取" {
          n1539 = stacked-sequence {
            seq-local: [_ w2533 _] -> [_ _ w2540]
            frame #0 {
              n1540 = local read "设备索引号"() -> (w2520:u16)
              n1541 = local read "CAN卡类型"() -> (w2521:u32)
              n1542 = local read "CAN端口"() -> (w2519:u16)
              n1543 = stacked-sequence {
                tunnel: w2521 -> [w2524 w2532]
                tunnel: w2520 -> [w2523 w2531]
                tunnel: w2519 -> [w2522 w2530]
                frame #0 {
                  n1544 = dll-call lib="PTH1abs FBluewave New EnergySVN_WorkAutoTest_TestStandtrunkAutoTest_TestStandDriverZlgCanBHN01è¯»ååæ°data\nkerneldlls\nusbcan.dll" fn="VCI_ClearBuffer"("DeviceType"=w2524, "DeviceInd"=w2523, "CANInd"=w2522) -> (error out=w2525:errorcluster)  [unwired: 4 in, 4 out]
                  n1545 = call <vilib>:"Clear Errors.vi"("error in (no error)"=w2525) -> ()  [unwired: 6 in, 1 out]
                }
                frame #1 {
                  w2529 = u8 137 ("命令")
                  w2528 = u32 1 ("命令序号")
                  n1546 = local read "从板板号"() -> (w2526:u8)
                  n1547 = local write "命令"(w2529) -> ()
                  n1548 = call "多帧发送机制(EV05).vi"("can卡类型"=w2532, "设备索引号"=w2531, "CAN端口"=w2530, "命令"=w2529, "板号"=w2526, "命令序号"=w2528, "输入数据"=dbl[] [0.0]) -> ()  [unwired: 2 in, 11 out]
                  n1549 = local write "命令序号"(w2528) -> ()
                }
              }
            }
            frame #1 {
              n1550 = while {
                tunnel: [w2534] -> w2533
                i -> [w2539]
                stop <- w2536 stop-if-true
                n1551 = global read "EV05全局变量1.vi" "写入超时"() -> (w2534:bool)
                n1552 = Greater Or Equal?(x=w2539, y=25) -> (x >= y?=w2537:bool)
                n1553 = Or(x=w2534, y=w2537) -> (x .or. y?=w2536:bool)
                n1554 = Wait Until Next ms Multiple(millisecond multiple=u32 100 ("毫秒倍数")) -> ()  [unwired: 1 out]
              }
            }
            frame #2 {
              n1555 = case shown="假" w2540 {
                frame False {
                  n1556 = control-ref of="结果"() -> (w2542:refnum<vi>)
                  n1557 = Concatenate Strings("项目软件版本" ("字符串"), "     读取失败" ("字符串")) -> (w2545:string)
                  n1558 = Build Array(w2545) -> (w2544:string[])
                  n1559 = call "表格编辑(版本读取).vi"("新元素/子数组"=w2544, "活动单元格:单元格背景色"=u32 16740749, "MCListbox引用句柄"=w2542) -> ()  [unwired: 9 out]
                }
                frame True {
                }
              }
              n1560 = call <vilib>:"Unset Busy.vi"() -> ()  [unwired: 2 in, 10 out]
            }
          }
        }
        frame "读取故障状态" {
          n1561 = stacked-sequence {
            seq-local: [_ w2571 _] -> [_ _ w2578]
            frame #0 {
              n1562 = local read "设备索引号"() -> (w2548:u16)
              n1563 = local read "CAN卡类型"() -> (w2549:u32)
              n1564 = local read "CAN端口"() -> (w2547:u16)
              n1565 = stacked-sequence {
                tunnel: w2549 -> [w2552 w2561]
                tunnel: w2548 -> [w2551 w2560]
                tunnel: w2547 -> [w2550 w2559]
                frame #0 {
                  n1566 = dll-call lib="PTH1abs FBluewave New EnergySVN_WorkAutoTest_TestStandtrunkAutoTest_TestStandDriverZlgCanBHN01è¯»ååæ°data\nkerneldlls\nusbcan.dll" fn="VCI_ClearBuffer"("DeviceType"=w2552, "DeviceInd"=w2551, "CANInd"=w2550) -> (error out=w2553:errorcluster)  [unwired: 4 in, 4 out]
                  n1567 = call <vilib>:"Clear Errors.vi"("error in (no error)"=w2553) -> ()  [unwired: 6 in, 1 out]
                }
                frame #1 {
                  n1568 = local read "从板板号 2"() -> (w2554:u8)
                  n1569 = case shown="1..30" w2554 {
                    tunnel: [u8 133 ("命令") u8 4 ("命令")] -> w2558
                    frame 0, Default {
                    }
                    frame 1..30 {
                    }
                  }
                  n1570 = local read "状态选择"() -> (w2556:T19)
                  n1571 = local write "命令"(w2558) -> ()
                  n1572 = case shown="\"预充电故障,继电器驱动故障\"" w2556 {
                    tunnel: [1 2 3 4 5 6 7] -> w2555
                    frame "电压,内总电压,外总电压,温度,电流,绝缘,系统时钟,充电均衡,放电均衡", Default {
                    }
                    frame "CPU,CPU内部EE存储器,CPU内部FLASH,内部EE存储器,45db存储器" {
                    }
                    frame "CAN检测故障" {
                    }
                    frame "软件故障" {
                    }
                    frame "RS485,RS232检测故障" {
                    }
                    frame "DI,DO,AI,AO检测故障" {
                    }
                    frame "预充电故障,继电器驱动故障" {
                    }
                  }
                  n1573 = call "多帧发送机制(EV05).vi"("can卡类型"=w2561, "设备索引号"=w2560, "CAN端口"=w2559, "命令"=w2558, "板号"=w2554, "命令序号"=w2555, "输入数据"=dbl[] [0.0]) -> ()  [unwired: 2 in, 11 out]
                  n1574 = local write "命令序号"(w2555) -> ()
                }
              }
            }
            frame #1 {
              n1575 = while {
                tunnel: [w2572] -> w2571
                i -> [w2577]
                stop <- w2574 stop-if-true
                n1576 = global read "EV05全局变量1.vi" "写入超时"() -> (w2572:bool)
                n1577 = Greater Or Equal?(x=w2577, y=25) -> (x >= y?=w2575:bool)
                n1578 = Or(x=w2572, y=w2575) -> (x .or. y?=w2574:bool)
